vi "SubVI_Read_PHD_FromSIS_ver2.4.vi"(7 "file path (dialog if empty)":path, 8 "Nominal m/z for SIS hist finding\nComma separated":string, 9 "MAX Event Rate":dbl=0.1 format="%#_13g", 10 "MIN Event Rate":dbl=0.005 format="%#_13g", 11 "Filter SIS by m/z?":bool) -> (0 "PHDHist":T2(graph), 1 "Average SIS from Filtered Data":cluster{dbl[], dbl[]}(graph), 2 "SIS Data":T1, 3 "Mean_mVns":dbl, 4 "Median_mVns":dbl, 5 "PHDValues":dbl[](array[numeric]))   [LabVIEW 2018]
uses:
  <vilib>/Analysis/NI_AALPro.lvlib
  <vilib>/Analysis/NI_AALBase.lvlib
panel:
  out "FWHM":dbl
  out "Max":dbl
  out "PulseHeightRes":dbl
  out "lowercase file extension":string
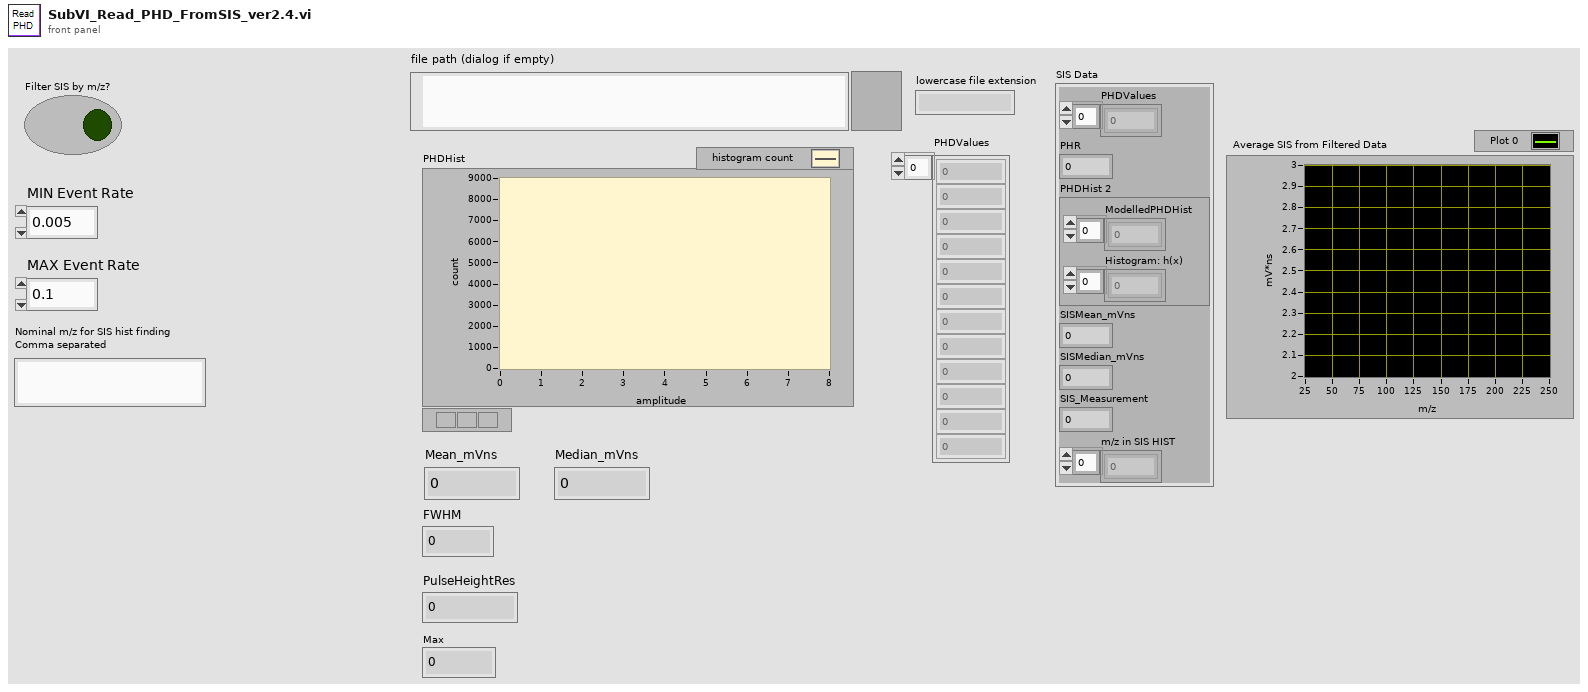
[diagram p1: front panel]
types:
  T1 = cluster{"PHDValues":dbl[], "PHR":dbl, "PHDHist 2":cluster{"ModelledPHDHist":dbl[], "Histogram: h(x)":i32[]}, "SISMean_mVns":dbl, "SISMedian_mVns":dbl, "SIS_Measurement":dbl, "m/z in SIS HIST":dbl[]}
  T2 = cluster{"X Values":dbl[], "Histogram: h(x)":i32[]}
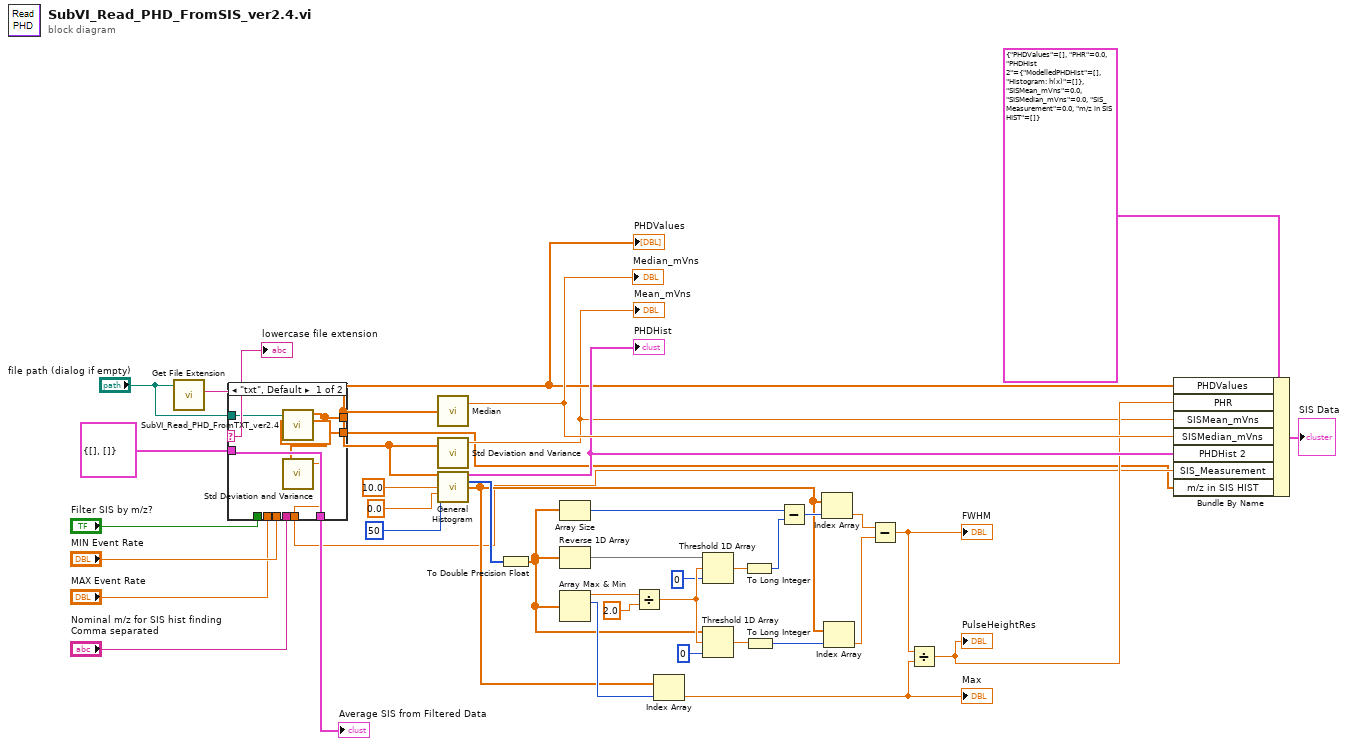
[diagram p0: block diagram]
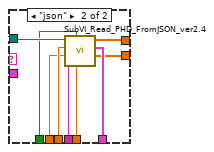
[diagram p2: hidden frame]
diagram:
  n1 = call <vilib>:"Get File Extension.vi"("file"="file path (dialog if empty)") -> ("lowercase file extension"=w33:string)  [unwired: 6 in, 4 out]
  "lowercase file extension" <- w33
  n2 = case shown="\"txt\", Default" w33 {
    tunnel: "file path (dialog if empty)" -> [w45 w54]
    tunnel: [w43 w53] -> w31
    tunnel: [w44 w52] -> w9
    tunnel: cluster{dbl[], dbl[]} {[], []} ("Average SIS from Filtered Data") -> [w44 _]
    tunnel: "MIN Event Rate" -> [_ w51]
    tunnel: "MAX Event Rate" -> [_ w50]
    tunnel: "Nominal m/z for SIS hist finding\nComma separated" -> [_ w49]
    tunnel: "Filter SIS by m/z?" -> [_ w48]
    tunnel: [w42 w47] -> w4
    tunnel: [dbl[] [] ("m/z in SIS Hist") w46] -> w2
    frame "txt", Default {
      n3 = call "SubVI_Read_PHD_FromTXT_ver2.4.vi"("file path (dialog if empty)"=w45) -> ("PHDValues"=w43:dbl[])  [unwired: 10 in]
      n4 = call <vilib>:"Std Deviation and Variance.vi"("X"=w43) -> ("mean"=w42:dbl)  [unwired: 1 in, 2 out]
    }
    frame "json" {
      n5 = call "SubVI_Read_PHD_FromJSON_ver2.4.vi"("Filter SIS by m/z?"=w48, "Nominal m/z for SIS hist finding\nComma separated"=w49, "MAX Event Rate"=w50, "MIN Event Rate"=w51, "file (use dialog)"=w54) -> ("m/z in SIS Hist"=w46:dbl[], "Average SIS from Filtered Data"=w52:cluster{dbl[], dbl[]}, "Filtered SIS Hist in mV-ns"=w53:dbl[], "AverageSis"=w47:dbl)  [unwired: 2 in]
    }
  }
  "PHDValues" <- w31
  "Average SIS from Filtered Data" <- w9
  n6 = call <vilib>:"Median.vi"("X"=w31) -> ("median"=w38:dbl)  [unwired: 1 out]
  "Median_mVns" <- w38
  n7 = call <vilib>:"Std Deviation and Variance.vi"("X"=w31) -> ("mean"=w3:dbl)  [unwired: 1 in, 2 out]
  "Mean_mVns" <- w3
  n8 = call <vilib>:"General Histogram.vi"("X"=w31, "max"=10.0, "min"=0.0, "# bins"=50) -> ("Histogram Graph"=w37:T2, "Histogram"=w40:i32[], "Axis"=w12:dbl[])  [unwired: 7 in, 2 out]
  "PHDHist" <- w37
  n9 = To Double Precision Float(number=w40) -> (double precision float=w13:dbl[])
  n10 = Array Size(array=w13) -> (size(s)=w19:i32)
  n11 = Reverse 1D Array(array=w13) -> (reversed array=w22:dbl[])
  n12 = Array Max & Min(array=w13) -> (max value=w16:dbl, max index (indices)=w18:i32)  [unwired: 2 out]
  n13 = Divide(x=w16, y=2.0) -> (x/y=w23:dbl)
  n14 = Index Array(array=w12, index=w18) -> (element=w14:dbl)
  "Max" <- w14
  n15 = Threshold 1D Array(1:0 ("start index (0)"), 2:w23, 3:w22) -> (0:w26:dbl)
  n16 = Threshold 1D Array(1:0 ("start index (0)"), 2:w23, 3:w13) -> (0:w28:dbl)
  n17 = To Long Integer(number=w26) -> (32bit integer=w20:i32)
  n18 = To Long Integer(number=w28) -> (32bit integer=w27:i32)
  n19 = Subtract(x=w19, y=w20) -> (x-y=w15:i32)
  n20 = Index Array(array=w12, index=w15) -> (element=w25:dbl)
  n21 = Index Array(array=w12, index=w27) -> (element=w24:dbl)
  n22 = Subtract(x=w25, y=w24) -> (x-y=w17:dbl)
  "FWHM" <- w17
  n23 = Divide(x=w17, y=w14) -> (x/y=w11:dbl)
  "PulseHeightRes" <- w11
  n24 = Bundle By Name(cluster=T1 {"PHDValues"=[], "PHR"=0.0, "PHDHist 2"={"ModelledPHDHist"=[], "Histogram: h(x)"=[]}, "SISMean_mVns"=0.0, "SISMedian_mVns"=0.0, "SIS_Measurement"=0.0, "m/z in SIS HIST"=[]} ("input cluster"), "PHDValues"=w31, "PHR"=w11, "SISMean_mVns"=w3, "SISMedian_mVns"=w38, "PHDHist 2"=w37, "SIS_Measurement"=w4, "m/z in SIS HIST"=w2) -> (→"SIS Data":T1)
